vi "UDP Data Link - Pages - Main Page.vi"(8 "error in (no error)":errorcluster, 11 "Node Ptr":T1 format="%.0x") -> (0 "error out":errorcluster)   [LabVIEW 2015, in "UDP Data Link System Explorer.lvlib"]
uses:
  UDP Data Link System Explorer.lvlib
  <vilib>/NI Veristand/Custom Device API/Custom Device Item Ref.ctl
  TypeDefs/UDP Data Link - TypeDefs - Main Page References.ctl
  Shared/UDP Data Link Global.vi
  <vilib>/NI Veristand/Custom Device API/Set Item Property (String).vi
  <vilib>/NI Veristand/Custom Device API/Set Item Property (Boolean).vi
  <vilib>/NI Veristand/Custom Device API/Set Item Property (U16).vi
  <vilib>/NI Veristand/Custom Device API/Set Item Property (I32).vi
  <vilib>/NI Veristand/Custom Device API/Set Item Property (Dependent Node Pointer).vi
  <vilib>/NI Veristand/Custom Device API/Set Item Property (Path).vi
  <vilib>/NI Veristand/Custom Device API/Custom Device API.lvlib
  Shared/UDP Data Link Shared.lvlib
  <vilib>/NI Veristand/Custom Device Tools/Custom Device Utility Library/Custom Device Utility Library.lvlib
panel:
  in  "Export Path":path
  in  "Export to File on Save":bool
  in  "Header 3":cluster{"Section Name":string}={"Section Name"="Custom Device Item Settings"}
  in  "Decimation":i32
  in  "Auto-Assign Local NIC":bool
  in  "Select Time-Stamp Channel":bool
  out "Timestamp Channel":string
  in  "Port":u16
  in  "IP Address of Remote Machine":string
  in  "IP Address of Local NIC":string
  in  "Header":cluster{"Section Name":string}={"Section Name"="Custom Device Item Settings"}
  in  "Name":string
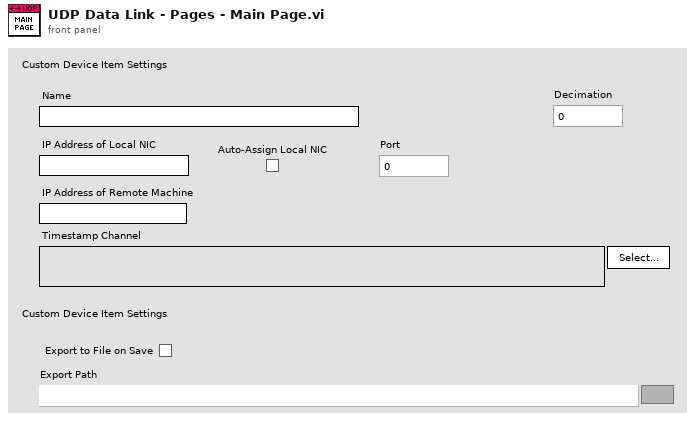
[diagram p1: front panel]
types:
  T1 = typedef "Custom Device API.lvlib/Custom Device Item Ref.ctl" = u64
  T2 = typedef "UDP Data Link System Explorer.lvlib/UDP Data Link - TypeDefs - Main Page References.ctl" = cluster{"Name":refnum<vi>, "Decimation":refnum<vi>, "IP Address of Local NIC":refnum<vi>, "Auto-Assign Local NIC":refnum<vi>, "Port":refnum<vi>, "IP Address of Remote Machine":refnum<vi>, "Timestamp Channel":refnum<vi>, "Export Path":refnum<vi>, "Export to File on Save":refnum<vi>}
  T3 = enum8{"Enabled", "Disabled", "Disabled and Grayed Out"}
  T4 = typedef "Custom Device API.lvlib/Custom Device Commands.ctl" = enum16{"Default", "Item renamed", "Shutdown", "Dynamic button pressed"}
  T5 = typedef "Custom Device API.lvlib/Custom Device Item Info.ctl" = cluster{"Name":string, "Is Channel":bool, "GUID":string, "Is Waveform":bool}
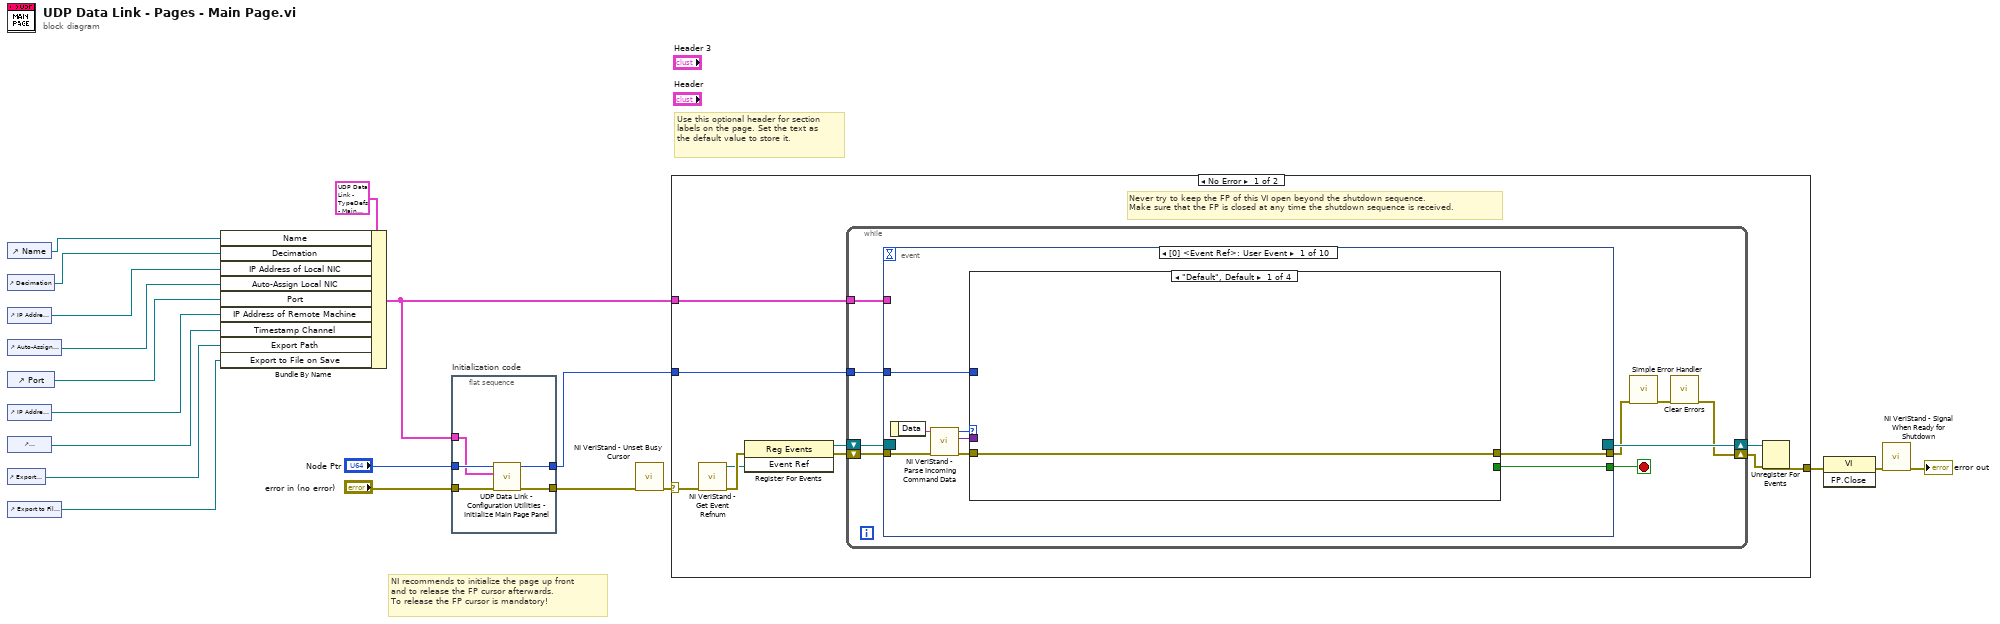
[diagram p0: block diagram]
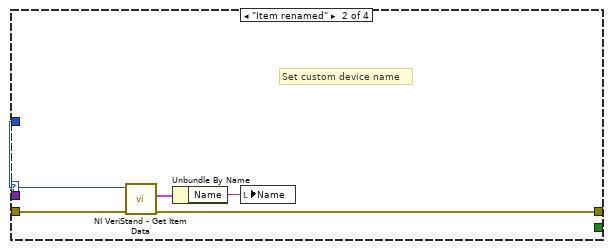
[diagram p2: hidden frame]
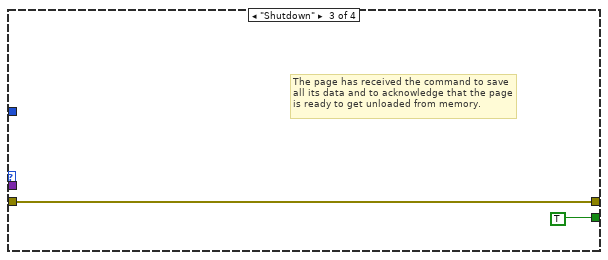
[diagram p3: hidden frame]
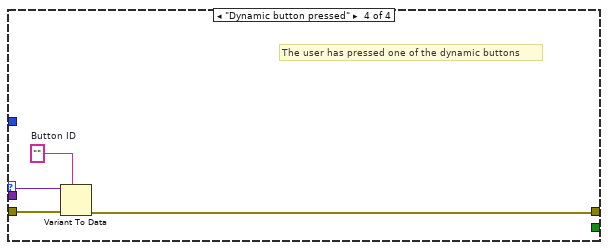
[diagram p4: hidden frame]
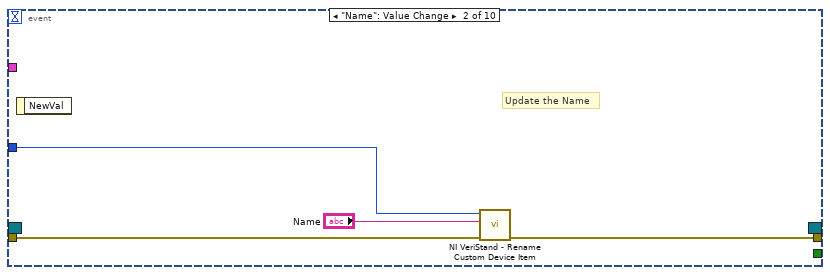
[diagram p5: hidden frame]
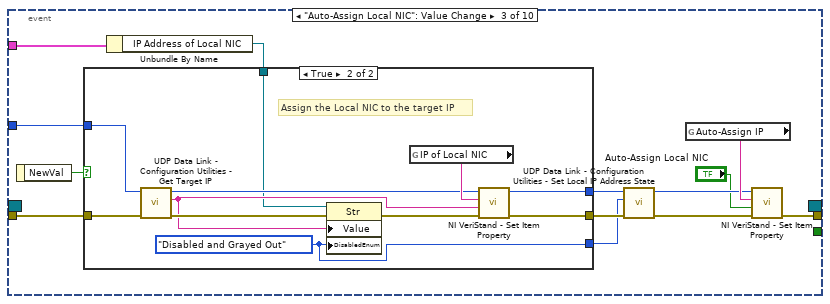
[diagram p6: hidden frame]
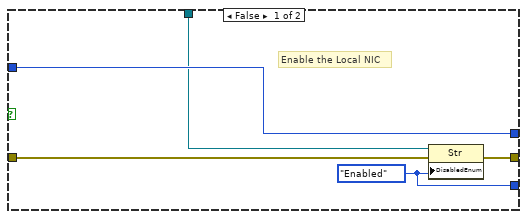
[diagram p7: hidden frame]
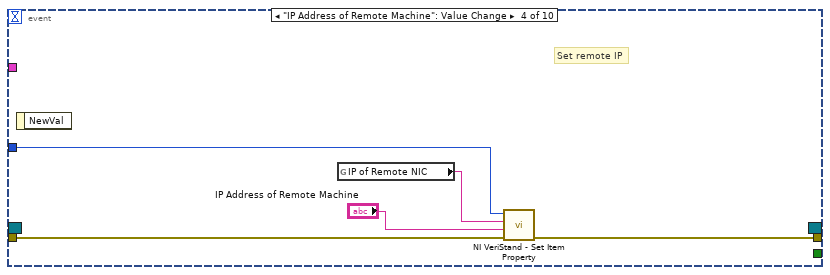
[diagram p8: hidden frame]
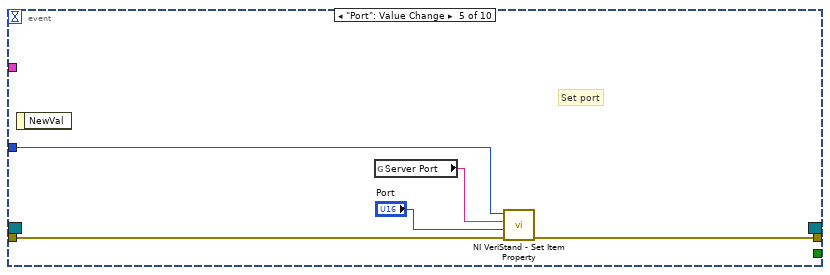
[diagram p9: hidden frame]
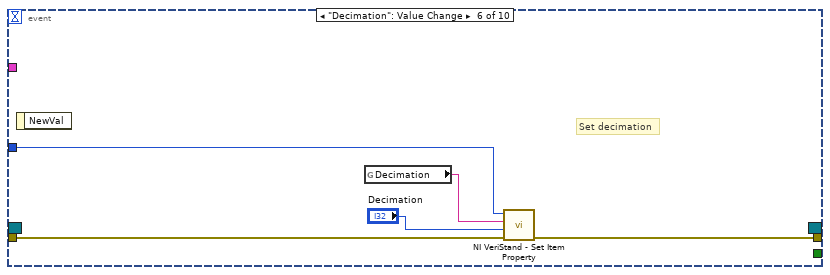
[diagram p10: hidden frame]
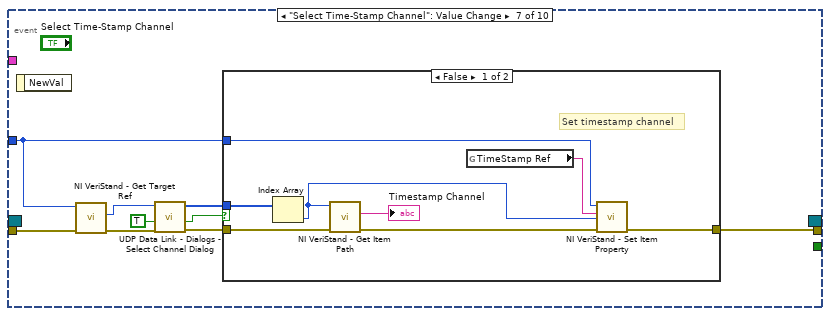
[diagram p11: hidden frame]
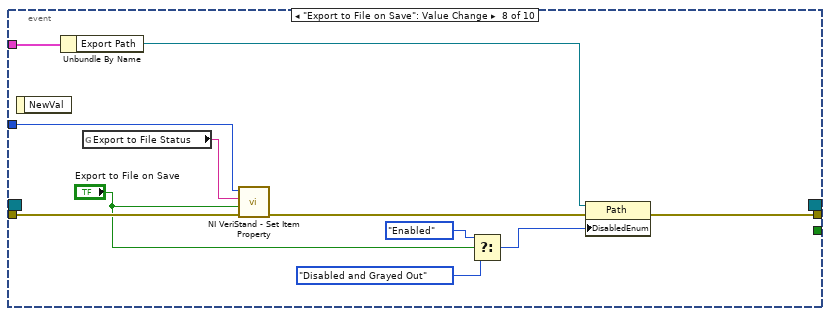
[diagram p13: hidden frame]
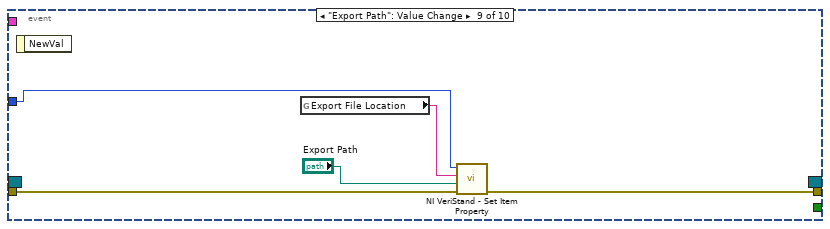
[diagram p14: hidden frame]
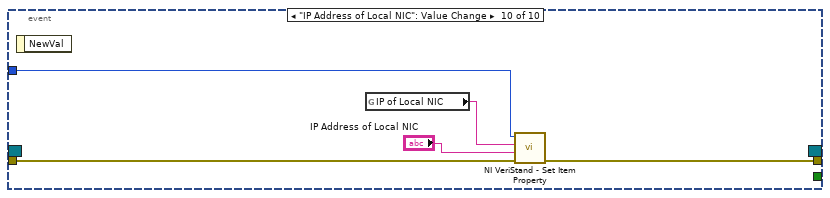
[diagram p15: hidden frame]
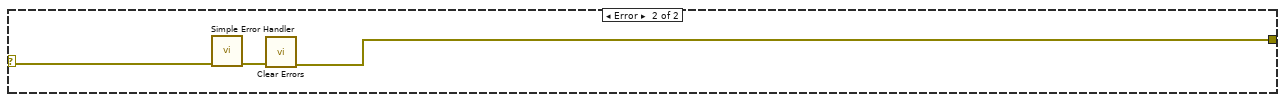
[diagram p16: hidden frame]
diagram:
  # "Use this optional header for section labels on the page. Set the text as the default value to store it."
  # "NI recommends to initialize the page up front\nand to release the FP cursor afterwards.\nTo release the FP cursor is mandatory!"
  n1 = control-ref of="Name"() -> (w10:refnum<vi>)
  n2 = control-ref of="Decimation"() -> (w9:refnum<vi>)
  n3 = control-ref of="IP Address of Local NIC"() -> (w8:refnum<vi>)
  n4 = control-ref of="Auto-Assign Local NIC"() -> (w7:refnum<vi>)
  n5 = control-ref of="Port"() -> (w6:refnum<vi>)
  n6 = control-ref of="IP Address of Remote Machine"() -> (w5:refnum<vi>)
  n7 = control-ref of="Timestamp Channel"() -> (w4:refnum<vi>)
  n8 = control-ref of="Export Path"() -> (w3:refnum<vi>)
  n9 = control-ref of="Export to File on Save"() -> (w2:refnum<vi>)
  n10 = Bundle By Name(cluster=T2 {"Name"=refnum, "Decimation"=refnum, "IP Address of Local NIC"=refnum, "Auto-Assign Local NIC"=refnum, "Port"=refnum, "IP Address of Remote Machine"=refnum, "Timestamp Channel"=refnum, "Export Path"=refnum, "Export to File on Save"=refnum}, "Name"=w10, "Decimation"=w9, "IP Address of Local NIC"=w8, "Auto-Assign Local NIC"=w7, "Port"=w6, "IP Address of Remote Machine"=w5, "Timestamp Channel"=w4, "Export Path"=w3, "Export to File on Save"=w2) -> (w1:T2)
  n11 = flat-sequence "Initialization code" {
    tunnel: "error in (no error)" -> [w24]
    tunnel: "Node Ptr" -> [w23]
    tunnel: [w21] -> w15
    tunnel: [w22] -> w12
    tunnel: w1 -> [w20]
    frame #0 {
      n12 = call "UDP Data Link - Configuration Utilities - Initialize Main Page Panel.vi"("error in (no error)"=w24, "Main Page References"=w20, "Item Ref in"=w23) -> ("error out"=w21:errorcluster, "Item Ref out"=w22:T1)  [unwired: 7 in]
    }
  }
  n13 = call <vilib>:"NI VeriStand - Unset Busy Cursor.vi"("error in (no error)"=w15) -> ("error out"=w14:errorcluster)  [unwired: 10 out]
  n14 = case shown="No Error" w14 {
    selector: w14 -> [w26 w152]
    tunnel: [w31 w150] -> w19
    tunnel: w12 -> [w27 _]
    tunnel: w1 -> [w25 _]
    frame No Error {
      # "Never try to keep the FP of this VI open beyond the shutdown sequence.\nMake sure that the FP is closed at any time the shutdown sequence is received."
      n15 = call <vilib>:"NI VeriStand - Get Event Refnum.vi"("error in (no error)"=w26) -> ("error out"=w34:errorcluster, "Event Ref"=w30:refnum<user-event>)  [unwired: 9 out]
      n16 = register-events(error in=w34, w30) -> (reference out=w28:refnum<event-registration>, error out=w29:errorcluster)  [unwired: 1 in]
      n17 = while {
        tunnel: w27 -> [w39]
        shift-right: [w36] -> w32
        shift-left: w29 -> [w42]
        shift-right: [w43] -> w33
        shift-left: w28 -> [w41]
        tunnel: w25 -> [w35]
        stop <- w40 stop-if-true
        n18 = event shown="[0] <Event Ref>: User Event" {
          selector: w41 -> [_ _ _ _ _ _ _ _ _ _]
          dyn-events: [_ _ _ _ _ _ _ _ _ _] -> w43
          timeout: _ -> [_ _ _ _ _ _ _ _ _ _]
          tunnel: w42 -> [w51 w67 w74 w97 w103 w108 w119 w139 w143 w146]
          tunnel: [w47 _ _ _ _ _ _ _ _ _] -> w40
          tunnel: [w46 w66 w72 w96 w102 w107 w112 w130 w140 w145] -> w38
          tunnel: w39 -> [w45 w65 w79 w98 w104 w109 w113 w137 w141 w148]
          tunnel: w35 -> [_ _ w71 _ _ _ _ w133 _ _]
          event User Event {
            n19 = event-data() -> ("Data"=w50:string)  [unwired: 1 out]
            n20 = call <vilib>:"NI VeriStand - Parse Incoming Command Data.vi"("error in (no error)"=w51, "Incoming data"=w50) -> ("error out"=w49:errorcluster, "Outgoing data"=w44:variant, "Action"=w48:T4)  [unwired: 7 out]
            n21 = case shown="\"Default\", Default" w48 {
              tunnel: w49 -> [w52 w57 w58 w63]
              tunnel: [_ _ TRUE _] -> w47
              tunnel: [w52 w54 w58 w60] -> w46
              tunnel: w45 -> [_ w56 _ _]
              tunnel: w44 -> [_ _ _ w62]
              frame "Default", Default {
              }
              frame "Item renamed" {
                # "Set custom device name"
                n22 = call <vilib>:"NI VeriStand - Get Item Data.vi"("error in (no error)"=w57, "Item Ref in"=w56) -> ("error out"=w54:errorcluster, "Item Info"=w55:T5)  [unwired: 8 out]
                n23 = Unbundle By Name(w55) -> ("Name"=w53:string)
                n24 = local write "Name"(w53) -> ()
              }
              frame "Shutdown" {
                # "The page has received the command to save all its data and to acknowledge that the page is ready to get unloaded from memory."
              }
              frame "Dynamic button pressed" {
                w61 = ""  # Button ID
                # "The user has pressed one of the dynamic buttons"
                n25 = Variant To Data(error in=w63, type=w61, Variant=w62) -> (error out=w60:errorcluster)  [unwired: 1 out]
              }
            }
          }
          event "Name": Value Change {
            # "Update the Name"
            n26 = event-data() -> ()  [unwired: 2 out]
            n27 = call <vilib>:"NI VeriStand - Rename Custom Device Item.vi"("error in (no error)"=w67, "New Name"="Name", "Item Ref in"=w65) -> ("error out"=w66:errorcluster)  [unwired: 1 in, 7 out]
          }
          event "Auto-Assign Local NIC": Value Change {
            n28 = event-data() -> ("NewVal"=w80:bool)  [unwired: 1 out]
            n29 = Unbundle By Name(w71) -> ("IP Address of Local NIC"=w70:refnum<vi>)
            n30 = case shown="True" w80 {
              tunnel: w79 -> [w85 w94]
              tunnel: [w85 w93] -> w78
              tunnel: w74 -> [w84 w92]
              tunnel: [w83 w91] -> w73
              tunnel: w70 -> [w82 w87]
              tunnel: [w81 w86] -> w69
              frame False {
                w81 = T3."Enabled" ("Disabled")
                # "Enable the Local NIC"
                n31 = property class="Str"(reference=w82, error in=w84, "DisabledEnum"=w81) -> (error out=w83:errorcluster)  [unwired: 1 out]
              }
              frame True {
                w86 = T3."Disabled and Grayed Out" ("Disabled")
                # "Assign the Local NIC to the target IP"
                n32 = call "UDP Data Link - Configuration Utilities - Get Target IP.vi"("error in"=w92, "Item Ref in"=w94) -> ("error out"=w90:errorcluster, "IPAddress"=w88:string)  [unwired: 7 in, 1 out]
                n33 = property class="Str"(reference=w87, error in=w90, "Value"=w88, "DisabledEnum"=w86) -> (error out=w89:errorcluster)  [unwired: 1 out]
                n34 = global read "UDP Data Link Global.vi" "IP of Local NIC"() -> (w95:string)
                n35 = call-poly <vilib>:"NI VeriStand - Set Item Property.vi"("error in (no error)"=w89, "Value"=w88, "Property Name"=w95, "Item Ref in"=w94) -> ("error out"=w91:errorcluster, "Item Ref out"=w93:T1)  [unwired: 5 in, 1 out]
              }
            }
            n36 = call "UDP Data Link - Configuration Utilities - Set Local IP Address State.vi"("error in (no error)"=w73, "State"=w69, "Item Ref in"=w78) -> ("error out"=w68:errorcluster, "Item Ref out"=w76:T1)  [unwired: 7 in]
            n37 = global read "UDP Data Link Global.vi" "Auto-Assign IP"() -> (w77:string)
            n38 = call-poly <vilib>:"NI VeriStand - Set Item Property.vi"("error in (no error)"=w68, "Value"="Auto-Assign Local NIC", "Property Name"=w77, "Item Ref in"=w76) -> ("error out"=w72:errorcluster)  [unwired: 5 in, 2 out]
          }
          event "IP Address of Remote Machine": Value Change {
            # "Set remote IP"
            n39 = event-data() -> ()  [unwired: 2 out]
            n40 = global read "UDP Data Link Global.vi" "IP of Remote NIC"() -> (w100:string)
            n41 = call-poly <vilib>:"NI VeriStand - Set Item Property.vi"("error in (no error)"=w97, "Value"="IP Address of Remote Machine", "Property Name"=w100, "Item Ref in"=w98) -> ("error out"=w96:errorcluster)  [unwired: 5 in, 2 out]
          }
          event "Port": Value Change {
            # "Set port"
            n42 = event-data() -> ()  [unwired: 2 out]
            n43 = global read "UDP Data Link Global.vi" "Server Port"() -> (w105:string)
            n44 = call-poly <vilib>:"NI VeriStand - Set Item Property.vi"("error in (no error)"=w103, "Value"="Port", "Property Name"=w105, "Item Ref in"=w104) -> ("error out"=w102:errorcluster)  [unwired: 5 in, 2 out]
          }
          event "Decimation": Value Change {
            # "Set decimation"
            n45 = event-data() -> ()  [unwired: 2 out]
            n46 = global read "UDP Data Link Global.vi" "Decimation"() -> (w110:string)
            n47 = call-poly <vilib>:"NI VeriStand - Set Item Property.vi"("error in (no error)"=w108, "Value"="Decimation", "Property Name"=w110, "Item Ref in"=w109) -> ("error out"=w107:errorcluster)  [unwired: 5 in, 2 out]
          }
          event "Select Time-Stamp Channel": Value Change {
            n48 = event-data() -> ()  [unwired: 2 out]
            n49 = call <vilib>:"NI VeriStand - Get Target Ref.vi"("error in"=w119, "Item Ref in"=w113) -> ("error out"=w118:errorcluster, "Target Ref"=w111:T1)  [unwired: 6 in, 2 out]
            n50 = call "UDP Data Link - Dialogs - Select Channel Dialog.vi"("error in (no error)"=w118, "Allow Section Selection (F)"=TRUE, "Root Item Ref"=w111) -> ("error out"=w116:errorcluster, "Canceled"=w115:bool, "Selected Channel Refs"=w114:T1[])  [unwired: 6 in]
            n51 = case shown="False" w115 {
              tunnel: w116 -> [w122 w128]
              tunnel: w114 -> [w125 _]
              tunnel: w113 -> [w126 _]
              tunnel: [w120 w128] -> w112
              frame False {
                # "Set timestamp channel"
                n52 = Index Array(array=w125) -> (element=w124:T1)  [unwired: 1 in]
                n53 = call <vilib>:"NI VeriStand - Get Item Path.vi"("error in (no error)"=w122, "Item Ref in"=w124) -> ("error out"=w123:errorcluster, "Path"=→"Timestamp Channel":string)  [unwired: 6 in, 2 out]
                n54 = global read "UDP Data Link Global.vi" "TimeStamp Ref"() -> (w127:string)
                n55 = call-poly <vilib>:"NI VeriStand - Set Item Property.vi"("error in (no error)"=w123, "Dependent Node Ref"=w124, "Property Name"=w127, "Item Ref in"=w126) -> ("error out"=w120:errorcluster)  [unwired: 7 out]
              }
              frame True {
              }
            }
          }
          event "Export to File on Save": Value Change {
            n56 = event-data() -> ()  [unwired: 2 out]
            n57 = Unbundle By Name(w133) -> ("Export Path"=w129:refnum<vi>)
            n58 = global read "UDP Data Link Global.vi" "Export to File Status"() -> (w138:string)
            n59 = call-poly <vilib>:"NI VeriStand - Set Item Property.vi"("error in (no error)"=w139, "Value"="Export to File on Save", "Property Name"=w138, "Item Ref in"=w137) -> ("error out"=w132:errorcluster)  [unwired: 5 in, 2 out]
            n60 = Select(t=T3."Enabled" ("Disabled"), s="Export to File on Save", f=T3."Disabled and Grayed Out" ("Disabled")) -> (s? t:f=w131:T3)
            n61 = property class="Path"(reference=w129, error in=w132, "DisabledEnum"=w131) -> (error out=w130:errorcluster)  [unwired: 1 out]
          }
          event "Export Path": Value Change {
            n62 = event-data() -> ()  [unwired: 2 out]
            n63 = global read "UDP Data Link Global.vi" "Export File Location"() -> (w144:string)
            n64 = call-poly <vilib>:"NI VeriStand - Set Item Property.vi"("error in (no error)"=w143, "Value"="Export Path", "Property Name"=w144, "Item Ref in"=w141) -> ("error out"=w140:errorcluster)  [unwired: 5 in, 2 out]
          }
          event "IP Address of Local NIC": Value Change {
            n65 = event-data() -> ()  [unwired: 2 out]
            n66 = global read "UDP Data Link Global.vi" "IP of Local NIC"() -> (w149:string)
            n67 = call-poly <vilib>:"NI VeriStand - Set Item Property.vi"("error in (no error)"=w146, "Value"="IP Address of Local NIC", "Property Name"=w149, "Item Ref in"=w148) -> ("error out"=w145:errorcluster)  [unwired: 5 in, 2 out]
          }
        }
        n68 = call <vilib>:"Simple Error Handler.vi"("error in (no error)"=w38) -> ("error out"=w37:errorcluster)  [unwired: 1 in, 7 out]
        n69 = call <vilib>:"Clear Errors.vi"("error in (no error)"=w37) -> ("error out"=w36:errorcluster)  [unwired: 1 in, 5 out]
      }
      n70 = Unregister For Events(event registration refnum=w33, error in=w32) -> (error out=w31:errorcluster)
    }
    frame Error {
      n71 = call <vilib>:"Simple Error Handler.vi"("error in (no error)"=w152) -> ("error out"=w151:errorcluster)  [unwired: 1 in, 7 out]
      n72 = call <vilib>:"Clear Errors.vi"("error in (no error)"=w151) -> ("error out"=w150:errorcluster)  [unwired: 1 in, 5 out]
    }
  }
  n73 = invoke class="VI" method="FP.Close"(error in=w19) -> (error out=w18:errorcluster)  [unwired: 2 in, 2 out]
  n74 = call <vilib>:"NI VeriStand - Signal When Ready for Shutdown.vi"("error in (no error)"=w18) -> ("error out"=→"error out":errorcluster)  [unwired: 10 out]
